vi "DeleteWaveformBusName.vi"(8 "error in (no error)":errorcluster, 9 "Waveform in":waveform(sgl)) -> (0 "error out":errorcluster, 1 "Waveform out":waveform(sgl))   [LabVIEW 2017, in "McsaVirtualChannel.lvlib"]
uses:
  <vilib>/addons/InsightCM/Devices/Shared/Mcsa/McsaVirtualChannel/McsaVirtualChannel.lvlib
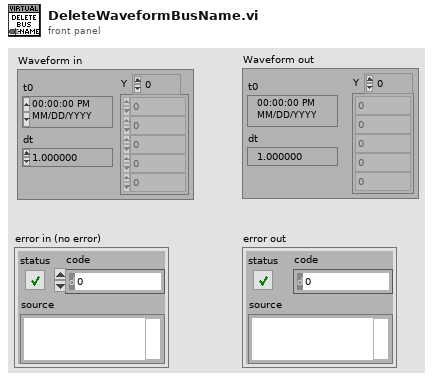
[diagram p1: front panel]
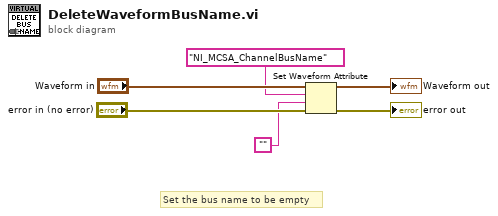
[diagram p0: block diagram]
diagram:
  # "Set the bus name to be empty"
  n1 = Set Waveform Attribute(4:"error in (no error)", 5:"", 6:"NI_MCSA_ChannelBusName" ("name"), 7:"Waveform in") -> (0:→"error out":errorcluster, 3:→"Waveform out":waveform(sgl))  [unwired: 1 out]
